vi "Memory.Pointer.Write.0D.U16.vi"(8 "error in (no error)":errorcluster, 9 "offset (0)":u64 format="%d bytes", 10 "value":u16, 11 "Pointer in":refnum<class "Memory.Pointer.lvclass">) -> (0 "error out":errorcluster, 1 "offset out":u64 format="%d bytes", 2 "value":u16, 3 "Pointer out":refnum<class "Memory.Pointer.lvclass">)   [LabVIEW 2016, in "Memory Manager.lvlib" / "Memory.Pointer.lvclass"]
doc: "Writes the provided <b>value</b> to the address specified by <b>pointer + offset</b>.\n\n<b>Note:</b> This VI is <b>safe</b>.\n\nSafe means that this function evaluates the size parameter of <b>pointer</b> to ensure that is inbounds of allocated memory before peforming a memory read/write. Reading/writing more data to a pointer than it has allocated can corrupt or crash LabVIEW."
uses:
  Memory.Pointer.lvclass
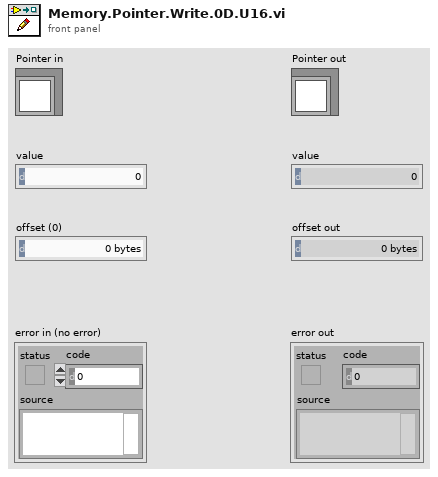
[diagram p1: front panel]
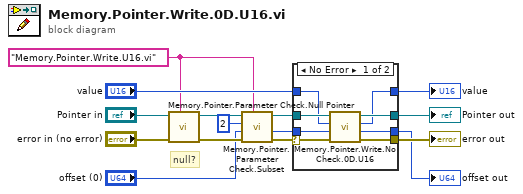
[diagram p0: block diagram]
diagram:
  w5 = "Memory.Pointer.Write.U16.vi" ("source vi name")
  # "null?"
  n1 = call "Memory.Pointer.Parameter Check.Null Pointer.vi"("source vi name"=w5, "error in (no error)"="error in (no error)", "Pointer in"="Pointer in") -> ("error out"=w6:errorcluster, "Pointer out"=w7:refnum<class "Memory.Pointer.lvclass">)  [unwired: 7 in]
  n2 = call "Memory.Pointer.Parameter Check.Subset.vi"("source vi name"=w5, "error in (no error)"=w6, "offset (0)"="offset (0)", "length"=u64 2 ("y"), "Pointer in"=w7) -> ("error out"=w14:errorcluster, "offset out"=w3:u64, "Pointer out"=w15:refnum<class "Memory.Pointer.lvclass">)  [unwired: 3 in, 1 out]
  n3 = case shown="No Error" w14 {
    selector: w14 -> [w19 w25]
    tunnel: w15 -> [w23 w27]
    tunnel: [w22 w27] -> w11
    tunnel: [w21 w26] -> w12
    tunnel: "value" -> [w20 w26]
    tunnel: [w18 w25] -> w13
    tunnel: w3 -> [w17 w24]
    tunnel: [w16 w24] -> w2
    frame No Error {
      n4 = call "Memory.Pointer.Write.No Check.0D.U16.vi"("error in (no error)"=w19, "offset (0)"=w17, "value"=w20, "Pointer in"=w23) -> ("error out"=w18:errorcluster, "offset out"=w16:u64, "value"=w21:u16, "Pointer out"=w22:refnum<class "Memory.Pointer.lvclass">)  [unwired: 4 in]
    }
    frame Error {
    }
  }
  "error out" <- w13
  "Pointer out" <- w11
  "value" <- w12
  "offset out" <- w2
